vi "Configure Controller.vi"(9 "WindowHandle":i32, 10 "Config File Path":path=path "MeasurementConfig.ini") -> (0 "error IO":errorcluster, 2 "Absolute Path":path, 4 "Canceled?":bool)   [LabVIEW 2016, in "Controller API.lvlib" / "Controller API.lvclass"]
uses:
  Controller API.lvclass
  MAL-Framework/user.lib/Common Components/Msmt Configuration/Controller Configuration.lvclass
  C:/Program Files (x86)/National Instruments/LabVIEW 2016/user.lib/Configuration Dialog Actor/Configuration.lvclass
  C:/Program Files (x86)/National Instruments/LabVIEW 2016/vi.lib/ActorFramework/Actor/Actor.lvclass
  <vilib>/ActorFramework/Message Queue/Message Queue.lvclass/Message Queue.ctl
  <vilib>/ActorFramework/LastAck/Last Ack.lvclass
  <vilib>/ActorFramework/Message Dequeuer/Message Dequeuer.lvclass/Message Dequeuer.ctl
  <vilib>/ActorFramework/LastAck/Last Ack.lvclass/Last Ack.ctl
  Extensible-Config-Dialog/Configuration.lvclass/Configuration.ctl
  <vilib>/ActorFramework/Message Priority Queue/Priority Dequeue.vi
  Extensible-Config-Dialog/Configuration.lvclass
  <vilib>/ActorFramework/Actor/Actor.lvclass
  <vilib>/ActorFramework/Message Queue/Message Queue.lvclass
  <vilib>/ActorFramework/Message Dequeuer/Message Dequeuer.lvclass
panel:
  out "Path to config file":path
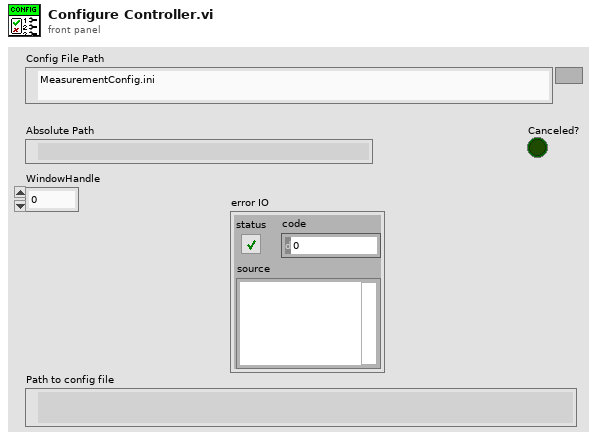
[diagram p1: front panel]
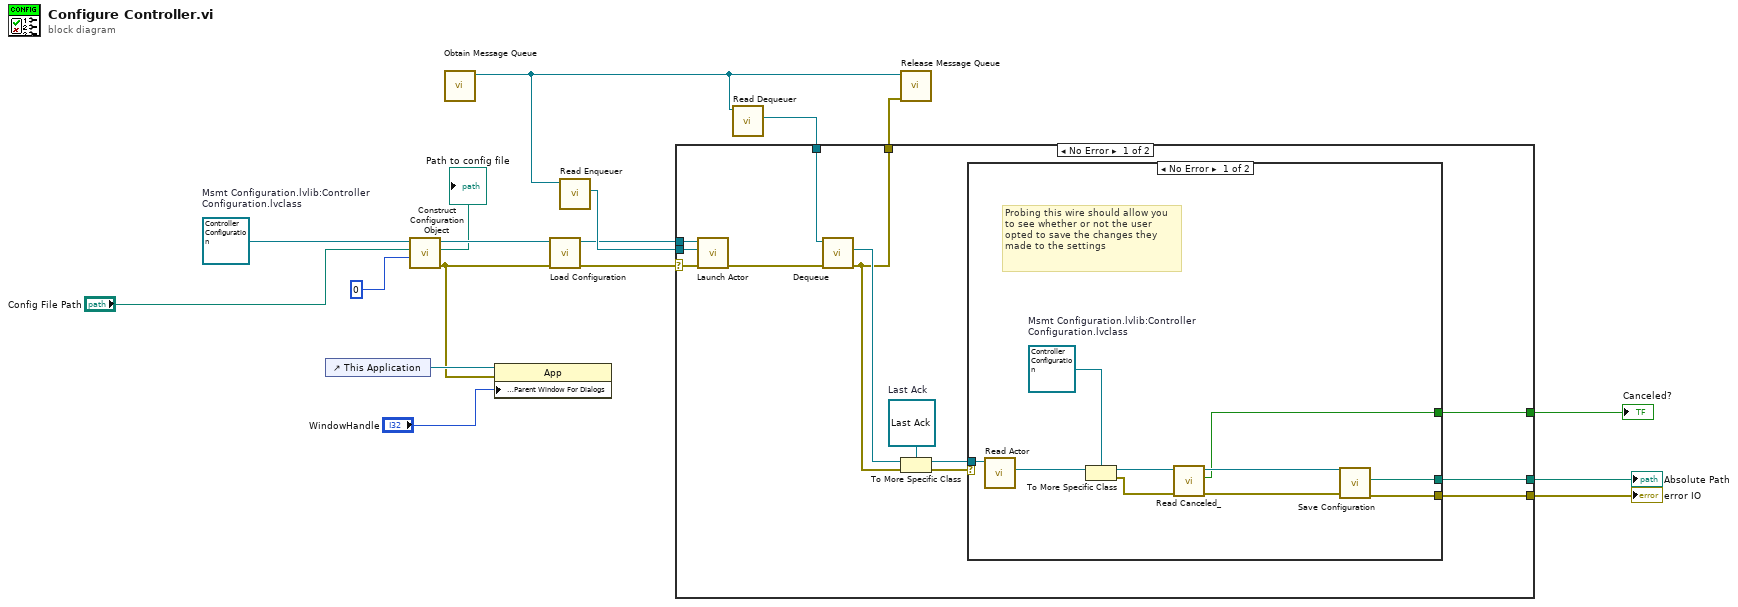
[diagram p0: block diagram]
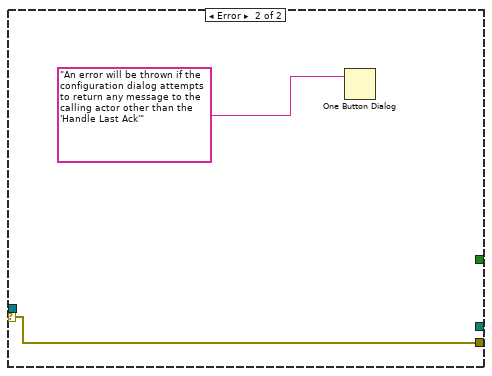
[diagram p2: hidden frame]
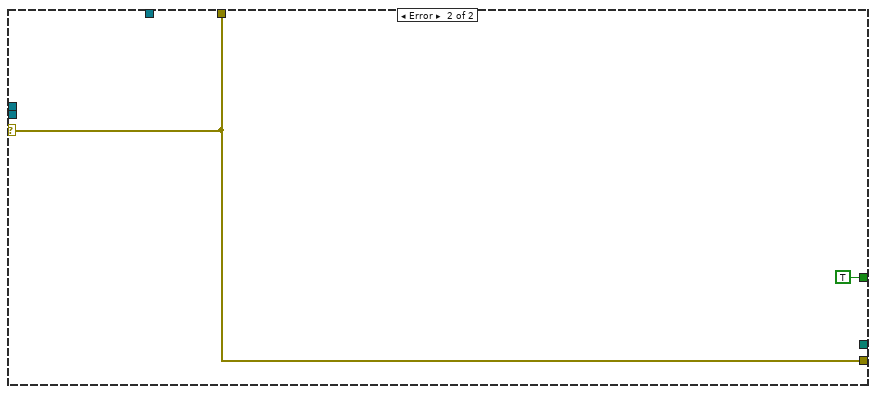
[diagram p3: hidden frame]
diagram:
  w17 = refnum<class "Controller Configuration.lvclass"> refnum  # Msmt Configuration.lvlib:Controller Configuration.lvclass
  n1 = control-ref of="This Application"() -> (w6:refnum<vi>)
  n2 = call "Construct Configuration Object.vi"("Initial Category Selection"=0, "Configuration File Path"="Config File Path", "Configuration in"=w17) -> ("error out"=w5:errorcluster, "Path to config file"=→"Path to config file":path, "Configuration out"=w15:refnum<class "Controller Configuration.lvclass">)  [unwired: 5 in, 1 out]
  n3 = call <vilib>:"Obtain Message Queue.vi"() -> ("Message Queue"=w13:refnum<class "Message Queue.lvclass">)  [unwired: 10 in, 1 out]
  n4 = property class="App"(reference=w6, error in=w5, "Application:Parent Window For Dialogs"="WindowHandle") -> ()  [unwired: 2 out]
  n5 = call "Load Configuration.vi"("error in (no error)"=w5, "Configuration in"=w15) -> ("error out"=w3:errorcluster, "Configuration out"=w8:refnum<class "Controller Configuration.lvclass">)  [unwired: 7 in, 1 out]
  n6 = call <vilib>:"Read Enqueuer.vi"("Message Queue"=w13) -> ("Message Enqueuer"=w14:refnum<class "Message Enqueuer.lvclass">)  [unwired: 10 in]
  n7 = call <vilib>:"Read Dequeuer.vi"("Message Queue"=w13) -> ("Message Dequeuer"=w12:refnum<class "Message Dequeuer.lvclass">)  [unwired: 10 in]
  n8 = case shown="No Error" w3 {
    selector: w3 -> [w18 w43]
    tunnel: w14 -> [w30 _]
    tunnel: w12 -> [w25 _]
    tunnel: [w23 w43] -> w11
    tunnel: [w22 w43] -> w10
    tunnel: [w21 _] -> w9
    tunnel: w8 -> [w20 _]
    tunnel: [w19 TRUE ("Canceled?")] -> w4
    frame No Error {
      w28 = refnum<class "Last Ack.lvclass"> refnum  # Last Ack
      n9 = call <vilib>:"Launch Actor.vi"("error in (no error)"=w18, "Actor-to-Caller Enqueuer"=w30, "Actor"=w20) -> ("error out"=w24:errorcluster)  [unwired: 7 in, 1 out]
      n10 = call <vilib>:"Dequeue.vi"("error in (no error)"=w24, "Message Dequeuer in"=w25) -> ("error out"=w23:errorcluster, "Message"=w29:refnum<class "Message.lvclass">)  [unwired: 5 in, 3 out]
      n11 = To More Specific Class(target class=w28, reference=w29, error in=w23) -> (specific class reference=w27:refnum<class "Last Ack.lvclass">, error out=w26:errorcluster)
      n12 = case shown="No Error" w26 {
        selector: w26 -> [_ w41]
        tunnel: w27 -> [w40 _]
        tunnel: [w38 w41] -> w22
        tunnel: [w37 _] -> w21
        tunnel: [w31 _] -> w19
        frame No Error {
          w36 = refnum<class "Controller Configuration.lvclass"> refnum  # Msmt Configuration.lvlib:Controller Configuration.lvclass
          # "Probing this wire should allow you to see whether or not the user opted to save the changes they made to the settings"
          n13 = call <vilib>:"Read Actor.vi"("Last Ack"=w40) -> ("Actor"=w39:refnum<class "Actor.lvclass">)  [unwired: 10 in]
          n14 = To More Specific Class(target class=w36, reference=w39) -> (specific class reference=w35:refnum<class "Controller Configuration.lvclass">, error out=w33:errorcluster)  [unwired: 1 in]
          n15 = call "Read Canceled_.vi"("error in (no error)"=w33, "Configuration in"=w35) -> ("error out"=w32:errorcluster, "Canceled?"=w31:bool, "Configuration out"=w34:refnum<class "Controller Configuration.lvclass">)  [unwired: 7 in]
          n16 = call "Save Configuration.vi"("error in (no error)"=w32, "Configuration in"=w34) -> ("error out"=w38:errorcluster, "file path"=w37:path)  [unwired: 7 in, 1 out]
        }
        frame Error {
          n17 = One Button Dialog(message="An error will be thrown if the configuration dialog attempts to return any message to the calling actor other than the 'Handle Last Ack'") -> ()  [unwired: 1 in, 1 out]
        }
      }
    }
    frame Error {
    }
  }
  "error IO" <- w10
  "Absolute Path" <- w9
  "Canceled?" <- w4
  n18 = call <vilib>:"Release Message Queue.vi"("error in (no error)"=w11, "Message Queue"=w13) -> ()  [unwired: 8 in, 2 out]
